vi "Cleanup.vi"(8 "error in (no error)":errorcluster, 11 "Node in":refnum<class "bt_WaitOn_Queue.lvclass">) -> (0 "error out":errorcluster, 3 "Node out":refnum<class "bt_WaitOn_Queue.lvclass">)   [LabVIEW 2021, in "BT.lvlib" / "bt_WaitOn_Queue.lvclass"]
uses:
  bt_WaitOn_Queue.lvclass
  bt_WaitOn_Queue.lvclass/bt_WaitOn_Queue.ctl
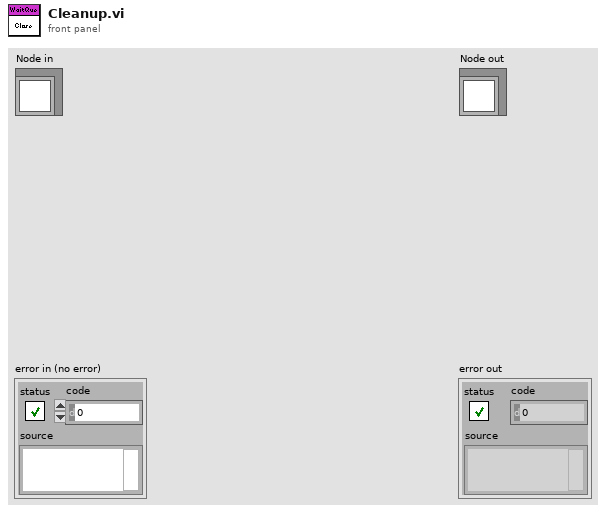
[diagram p1: front panel]
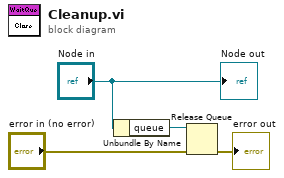
[diagram p0: block diagram]
diagram:
  n1 = Unbundle By Name("Node in") -> ("queue"=w1:refnum<queue>)
  n2 = Release Queue(queue=w1, error in (no error)="error in (no error)") -> (error out=→"error out":errorcluster)  [unwired: 1 in, 2 out]
  "Node out" <- "Node in"
